vi "Get Actual Speed.vi"(8 "error in":errorcluster, 10 "MCU Selector":T1, 11 "HSU MCU V2 Monitor CFG in":refnum<class "HSU MCU V2 Monitor CFG.lvclass">) -> (0 "error out":errorcluster, 2 "Speed":dbl format="%#_g rpm", 3 "HSU MCU V2 Monitor CFG out":refnum<class "HSU MCU V2 Monitor CFG.lvclass">)   [LabVIEW 2023, in "HSU MCU V2 Monitor CFG.lvclass"]
doc: "Speed of Motor in rpm"
uses:
  HSU MCU V2 Monitor CFG.lvclass
  HSU MCU V2 Monitor CFG.lvclass/HSU MCU V2 Monitor CFG.ctl
  Protocols/ICAN/ICAN.lvclass
  MCU Selector.ctl
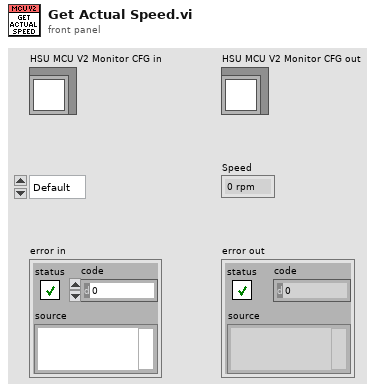
[diagram p1: front panel]
types:
  T1 = typedef "MCU Selector.ctl" = enum16{"Default", "MCU1", "MCU2", "MCU3", "MCU4", "MCU5", "MCU6", "MCU7", "MCU8"}
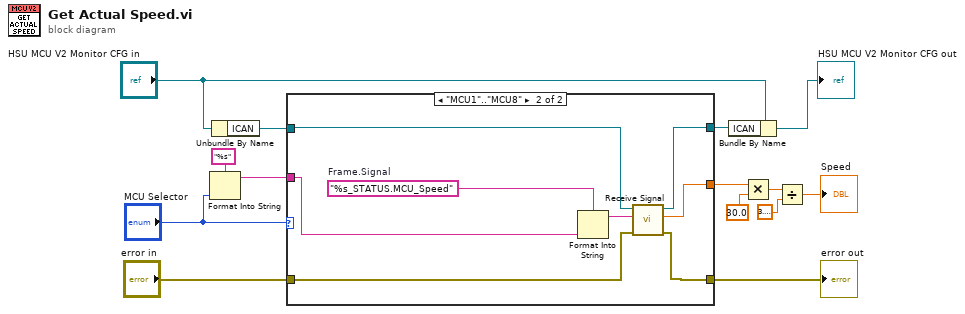
[diagram p0: block diagram]
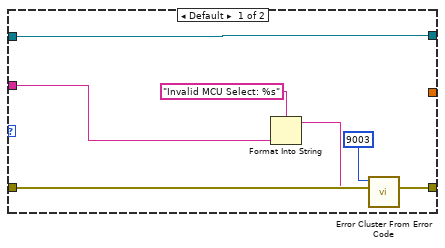
[diagram p2: hidden frame]
diagram:
  n1 = Format Into String(format string="%s", "MCU Selector") -> (resulting string=w13:string)  [unwired: 2 in, 1 out]
  n2 = Unbundle By Name("HSU MCU V2 Monitor CFG in") -> ("ICAN"=w12:refnum<class "ICAN.lvclass">)
  n3 = case shown="\"MCU1\"..\"MCU8\"" "MCU Selector" {
    tunnel: "error in" -> [w21 w27]
    tunnel: [w20 w26] -> w9
    tunnel: w13 -> [w16 w29]
    tunnel: w12 -> [w15 w28]
    tunnel: [w15 w25] -> w11
    tunnel: [_ w22] -> w5
    frame Default {
      n4 = Format Into String(format string="Invalid MCU Select: %s" ("error message (\"\")"), w16) -> (resulting string=w18:string)  [unwired: 2 in, 1 out]
      n5 = call <vilib>:"Error Cluster From Error Code.vi"("error in (no error)"=w21, "error message (\"\")"=w18, "error code (0)"=9003) -> ("error out"=w20:errorcluster)  [unwired: 6 in]
    }
    frame "MCU1".."MCU8" {
      w24 = "%s_STATUS.MCU_Speed"  # Frame.Signal
      n6 = Format Into String(format string=w24, w29) -> (resulting string=w23:string)  [unwired: 2 in, 1 out]
      n7 = call-dynamic "Receive Signal.vi"("error in"=w27, "Frame.Signal"=w23, "ICommunicate in"=w28) -> ("error out"=w26:errorcluster, "Value"=w22:dbl, "ICommunicate out"=w25:refnum<class "ICAN.lvclass">)  [unwired: 6 in]
    }
  }
  "error out" <- w9
  n8 = Bundle By Name(cluster="HSU MCU V2 Monitor CFG in", "ICAN"=w11) -> (→"HSU MCU V2 Monitor CFG out":refnum<class "HSU MCU V2 Monitor CFG.lvclass">)
  n9 = Multiply(x=w5, y=30.0) -> (x*y=w3:dbl)
  n10 = Divide(x=w3, y=3.141592653589793) -> (x/y=→"Speed":dbl)
